vi "Init.vi"(3 "Container State":T7, 4 "Previous State":variant, 5 "Previous Version":T6) -> (2 "Current State":T1)   [LabVIEW 2015, in "Interactive Graph.xctl"]
uses:
  Interactive Graph.xctl
  State.vi
  Persistent.ctl
  Plot.ctl
  EPhys/LV Source/Work Panel VIs/Typedefs/EPhysWork-Label Position.ctl
  Events.ctl
  Selection.ctl
  XRange.ctl
  YScale.ctl
  Cursor.ctl
  <vilib>/_xctls/Container State.ctl
  <vilib>/_xctls/Version.ctl
  <vilib>/_xctls/XControlSupport.lvlib
panel:
  in  "Default Indicator State":T1={"ref"=refnum, "actions"=[], "Persist"={"Scale"=1e-06, "Xrange"={"min"=0.0, "max"=10.0}}, "cursor"=FALSE, "prescale"=0.0, "palette"=[], "colIndex"=0, "to add"={"plot"={"X"=[], "Y"=[]}, "name"="", "Y0"=0.0, "color"=0, "Style"=enum."Normal", "labpos"={"Index"=0, "Xoff"=0.0, "Yoff"=0.0}, "visible"=FALSE, "cursor"=FALSE}, "Events"={"Selection"=refnum, "XRange"=refnum, "YScale"=refnum, "CursorPos"=refnum}, "selected"=0, "to show"={"Visible"=FALSE, "Start"=0, "Length"=0}, "maxplot"=0, "Y0"=[], "plotnum"=0}
  in  "Default Control State":T1={"ref"=refnum, "actions"=[], "Persist"={"Scale"=1e-06, "Xrange"={"min"=0.0, "max"=10.0}}, "cursor"=FALSE, "prescale"=0.0, "palette"=[], "colIndex"=0, "to add"={"plot"={"X"=[], "Y"=[]}, "name"="", "Y0"=0.0, "color"=0, "Style"=enum."Normal", "labpos"={"Index"=0, "Xoff"=0.0, "Yoff"=0.0}, "visible"=FALSE, "cursor"=FALSE}, "Events"={"Selection"=refnum, "XRange"=refnum, "YScale"=refnum, "CursorPos"=refnum}, "selected"=0, "to show"={"Visible"=FALSE, "Start"=0, "Length"=0}, "maxplot"=0, "Y0"=[], "plotnum"=0}
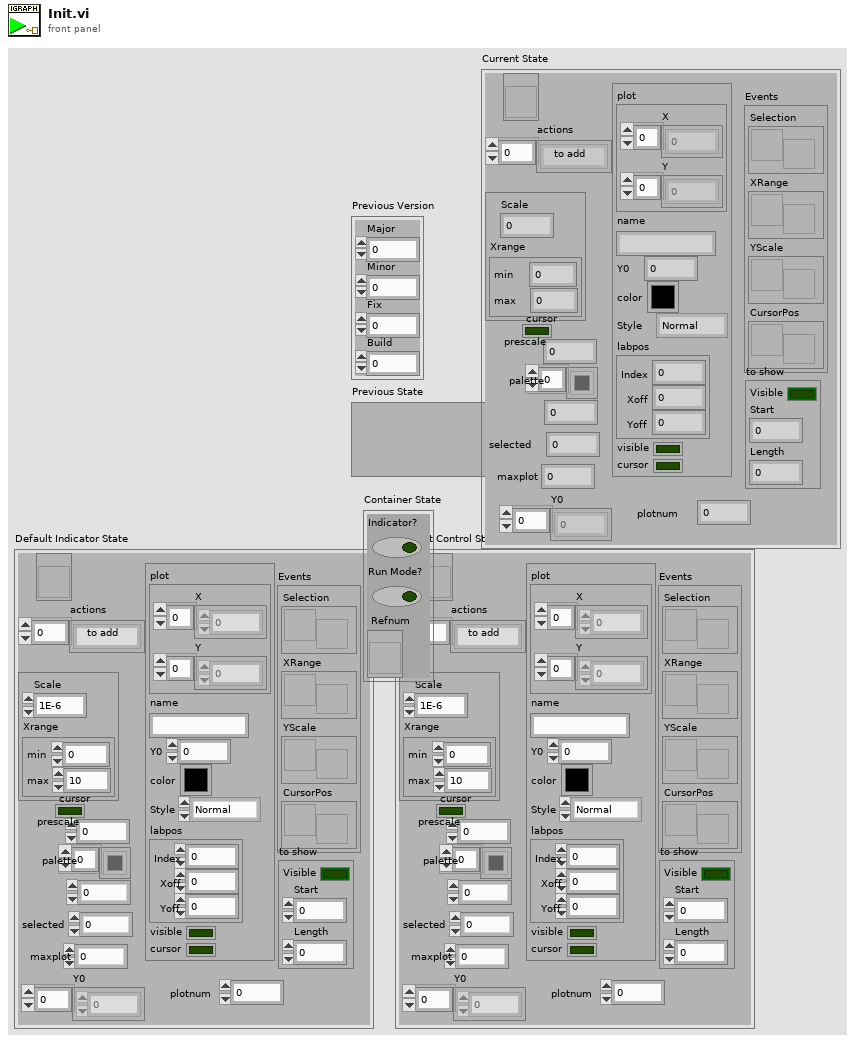
[diagram p1: front panel]
types:
  T1 = typedef "Interactive Graph.xctl/State.vi" = cluster{"ref":refnum<vi>, "actions":string[], "Persist":T2, "cursor":bool, "prescale":dbl, "palette":u32[], "colIndex":i32, "to add":T3, "Events":T5, "selected":i32, "to show":cluster{"Visible":bool, "Start":i32, "Length":i32}, "maxplot":i32, "Y0":dbl[], "plotnum":i32}
  T2 = typedef "Interactive Graph.xctl/Persistent.ctl" = cluster{"Scale":dbl, "Xrange":cluster{"min":dbl, "max":dbl}}
  T3 = typedef "Interactive Graph.xctl/Plot.ctl" = cluster{"plot":cluster{"X":dbl[], "Y":dbl[]}, "name":string, "Y0":dbl, "color":u32, "Style":enum16{"Normal", "Highlight", "Shadow"}, "labpos":T4, "visible":bool, "cursor":bool}
  T4 = typedef "EPhysWork-Label Position.ctl" = cluster{"Index":i32, "Xoff":dbl, "Yoff":dbl}
  T5 = typedef "Interactive Graph.xctl/Events.ctl" = cluster{"Selection":refnum<user-event>, "XRange":refnum<user-event>, "YScale":refnum<user-event>, "CursorPos":refnum<user-event>}
  T6 = typedef "XControlSupport.lvlib/Version.ctl" = cluster{"Major":u16, "Minor":u16, "Fix":u16, "Build":u16}
  T7 = typedef "XControlSupport.lvlib/Container State.ctl" = cluster{"Indicator?":bool, "Run Mode?":bool, " Refnum":refnum<vi>}
  T8 = enum16{"User", "Prism", "Kelly", "Dark2", "Sequential", "Hue"}
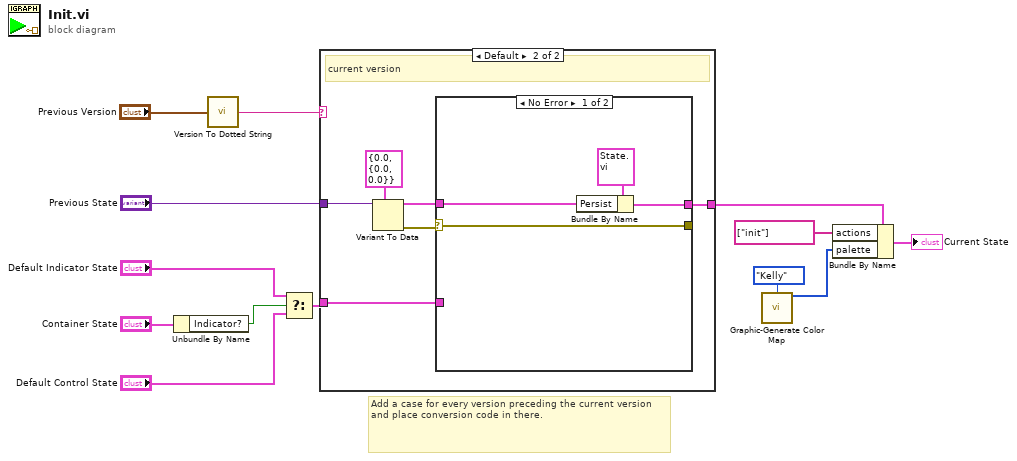
[diagram p0: block diagram]
diagram:
  # "Add a case for every version preceding the current version and place conversion code in there."
  n1 = Unbundle By Name("Container State") -> ("Indicator?"=w8:bool)
  n2 = call <vilib>:"Version To Dotted String.vi"("Version"="Previous Version") -> ("String Version"=w5:string)
  n3 = Select(t="Default Indicator State", s=w8, f="Default Control State") -> (s? t:f=w7:T1)
  n4 = case shown="Default" w5 {
    tunnel: "Previous State" -> [_ w16]
    tunnel: [w14 w17] -> w12
    tunnel: w7 -> [w14 w18]
    frame "0.0.0.0" {
      # "Just created, use default state"
    }
    frame Default {
      # "current version"
      n5 = Variant To Data(type=T2 {"Scale"=0.0, "Xrange"={"min"=0.0, "max"=0.0}} ("Persist"), Variant=w16) -> (data=w19:T2, error out=w20:errorcluster)  [unwired: 1 in]
      n6 = case shown="No Error" w20 {
        selector: w20 -> [w24 w25]
        tunnel: w19 -> [w22 _]
        tunnel: [w21 w26] -> w17
        tunnel: w18 -> [_ w26]
        tunnel: [w24 w25] -> _
        frame No Error {
          n7 = Bundle By Name(cluster=T1 {"ref"=refnum, "actions"=[], "Persist"={"Scale"=0.0, "Xrange"={"min"=0.0, "max"=0.0}}, "cursor"=FALSE, "prescale"=0.0, "palette"=[], "colIndex"=0, "to add"={"plot"={"X"=[], "Y"=[]}, "name"="", "Y0"=0.0, "color"=0, "Style"=enum."Normal", "labpos"={"Index"=0, "Xoff"=0.0, "Yoff"=0.0}, "visible"=FALSE, "cursor"=FALSE}, "Events"={"Selection"=refnum, "XRange"=refnum, "YScale"=refnum, "CursorPos"=refnum}, "selected"=0, "to show"={"Visible"=FALSE, "Start"=0, "Length"=0}, "maxplot"=0, "Y0"=[], "plotnum"=0} ("output cluster"), "Persist"=w22) -> (w21:T1)
        }
        frame Error {
          # "Error converting previously \nsaved state. Use default instead."
        }
      }
    }
  }
  n8 = call "Graphic-Generate Color Map.vi"("Map"=T8."Kelly") -> ("Colors"=w1:u32[])  [unwired: 14 in]
  n9 = Bundle By Name(cluster=w12, "actions"=string[] ["init"], "palette"=w1) -> (→"Current State":T1)
